vi "NO_NO_AutoNetwork.vi"(8 "error in (no error)":errorcluster) -> (0 "error out":errorcluster)   [LabVIEW 2023]
doc: "Network for Autonomous\n\nInputs:\n -- error in -- cluster\n\nOutputs:\n -- error in -- cluster"
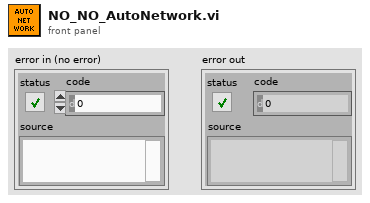
[diagram p1: front panel]
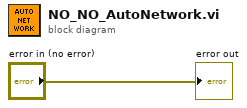
[diagram p0: block diagram]
diagram:
  "error out" <- "error in (no error)"
